vi "test_TCP_TCP Read.vi"(8 "error in (no error)":errorcluster, 11 "TestCase in":refnum<class "Ethernet Protocol Tests.lvclass">) -> (0 "error out":errorcluster, 3 "TestCase out":refnum<class "Ethernet Protocol Tests.lvclass">)   [LabVIEW 2019, in "Ethernet Protocol Tests.lvclass"]
uses:
  Ethernet Protocol Tests.lvclass
  ListenerVi/TCP/TCP.lvclass
  D:/GitRepository/niveristand-instrument-addon-classes/Source/Protocols/Tests/ListenerVi/Protocol Parent/Protocol Parent.lvclass
  ListenerVi/Listener.lvclass
  ListenerVi/TCP/TCP.lvclass/TCP.ctl
  ListenerVi/ListenerClassControls/Operation Ctl.ctl
  ListenerVi/Protocol Parent/Methods/Read Parameter.ctl
  <vilib>/addons/_JKI Toolkits/VI Tester/TestCase.llb/TestCase.lvclass
  ListenerVi/Protocol Parent/Protocol Parent.lvclass
  C:/Program Files (x86)/National Instruments/LabVIEW 2019/vi.lib/addons/_JKI Toolkits/VI Tester/TestCase.llb/TestCase.lvclass
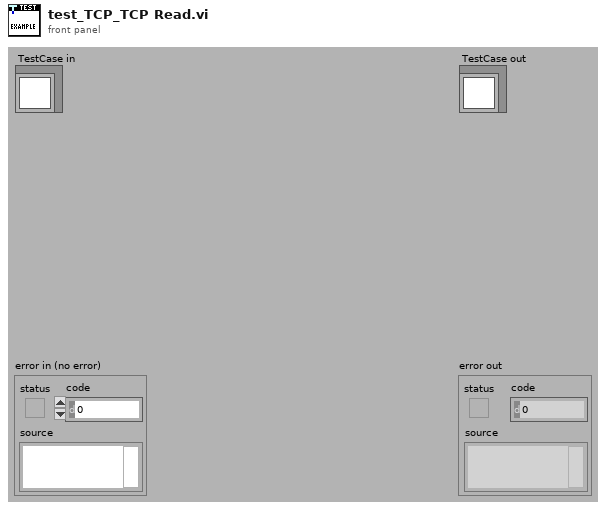
[diagram p1: front panel]
types:
  T1 = typedef "Localhost Protocols.lvlib/Protocol Parent.lvclass/Read Parameter.ctl" = cluster{"Wait Type":enum16{"Byte Count", "Wait sec"}, "Wait Value":dbl}
  T2 = typedef "Operation Ctl.ctl" = enum16{"Read", "Write"}
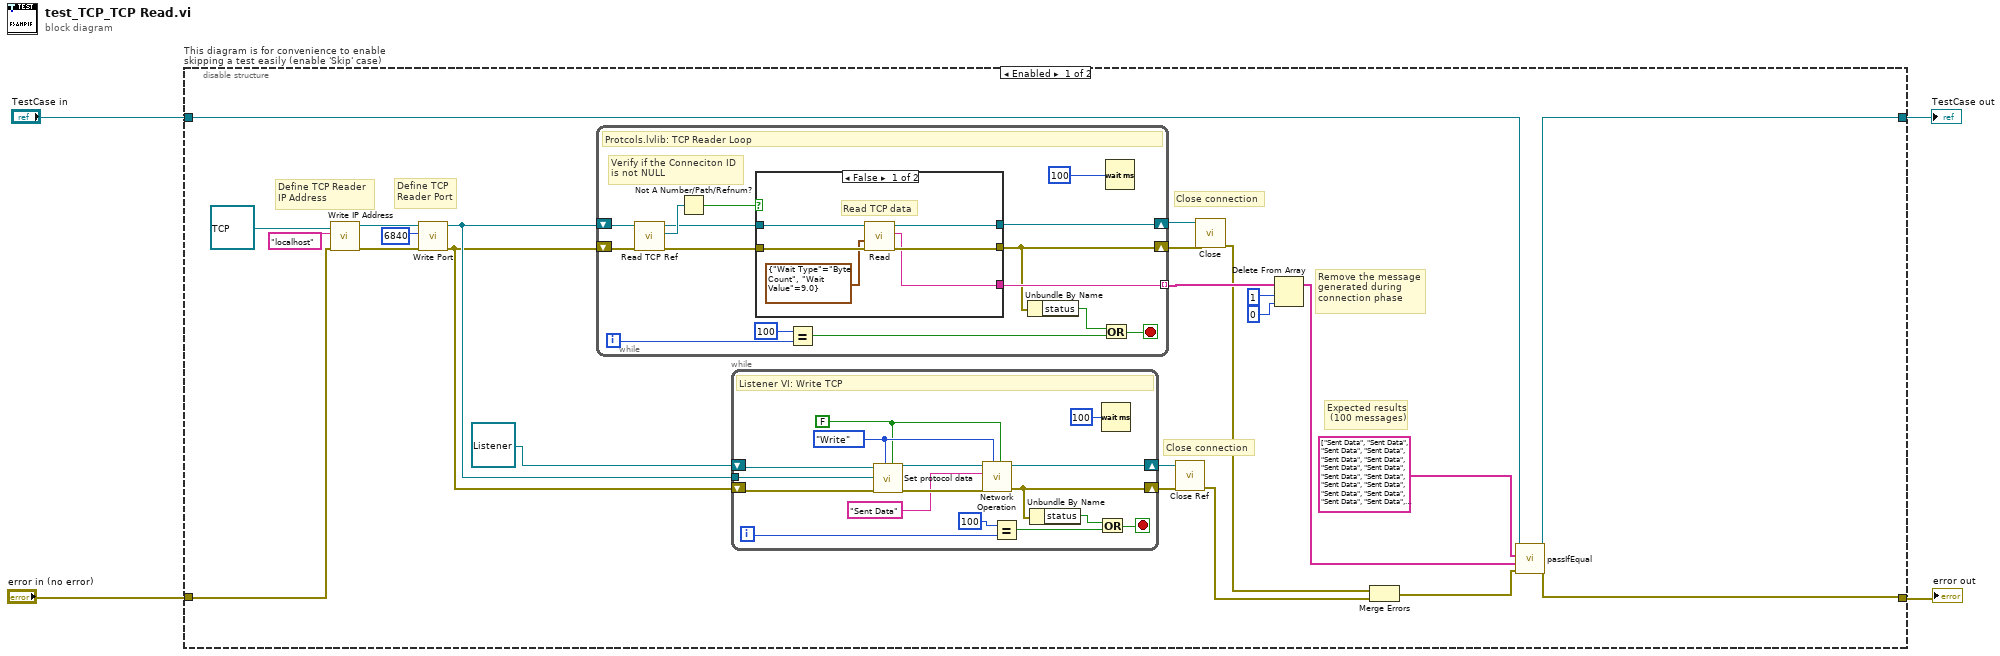
[diagram p0: block diagram]
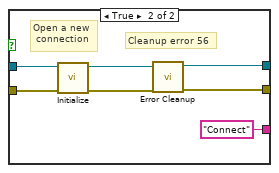
[diagram p2: hidden frame]
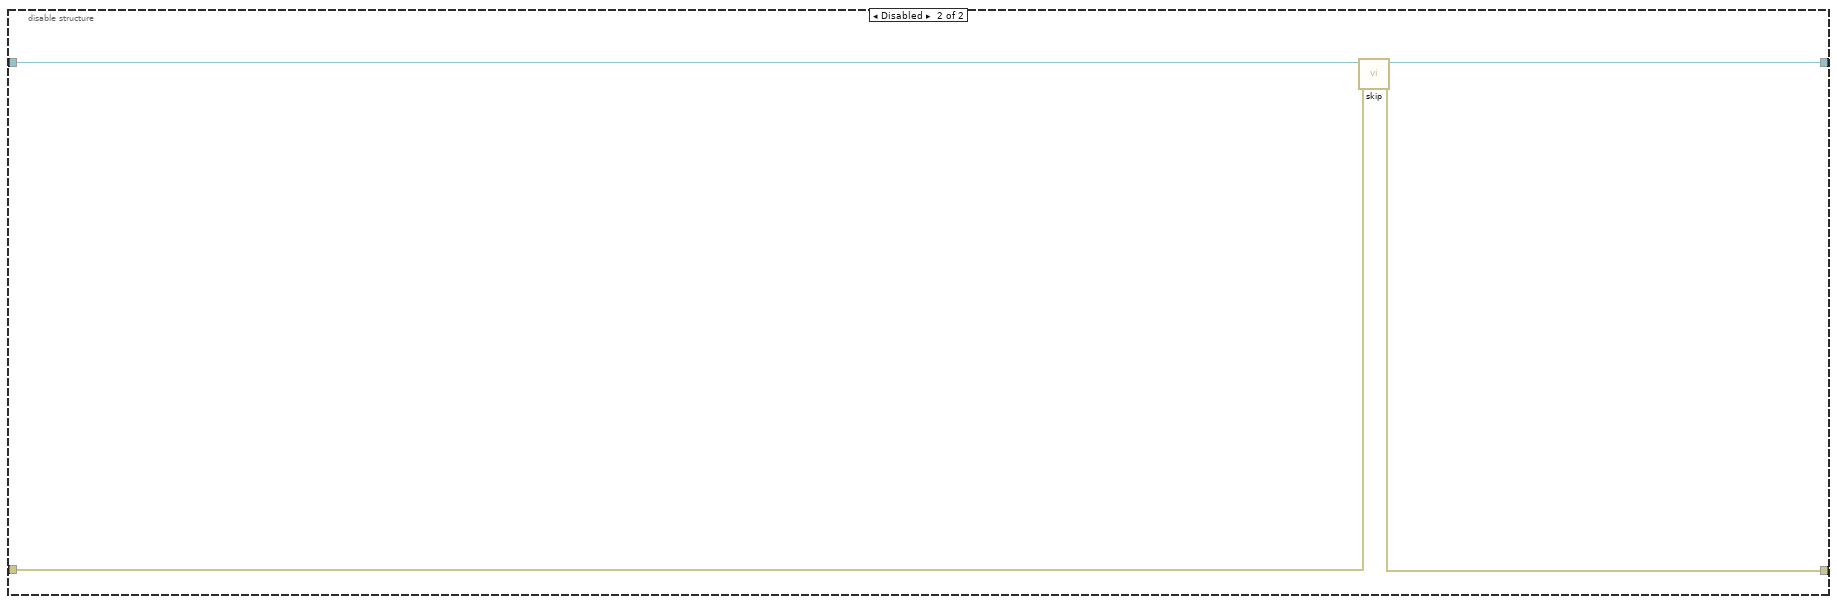
[diagram p3: hidden frame]
diagram:
  n1 = disable-structure "This diagram is for convenience to enable skipping a test easily (enable 'Skip' case)" shown="Enabled" {
    disable-tunnel: "TestCase in" -> [w28 w76]
    disable-tunnel: [w27 w74] -> w1
    disable-tunnel: [w26 w75] -> w3
    disable-tunnel: "error in (no error)" -> [w17 w73]
    frame Enabled {
      # "Close connection"
      # "Close connection"
      # "Remove the message\ngenerated during \nconnection phase"
      # "Expected results\n (100 messages)"
      # "Define TCP \nReader Port"
      # "Define TCP Reader \nIP Address"
      n2 = call "Write IP Address.vi"("error in (no error)"=w17, "IP Address"="localhost", "Ethernet in"=refnum<class "TCP.lvclass"> refnum ("Localhost Protocols.lvlib:TCP.lvclass")) -> ("error out"=w22:errorcluster, "Ethernet out"=w23:refnum<class "TCP.lvclass">)  [unwired: 7 in]
      n3 = call "Write Port.vi"("error in (no error)"=w22, "Port"=u16 6840, "Ethernet in"=w23) -> ("error out"=w18:errorcluster, "Ethernet out"=w20:refnum<class "TCP.lvclass">)  [unwired: 7 in]
      n4 = while {
        shift-right: [w49] -> w10
        shift-left: w18 -> [w59]
        shift-right: [w53] -> w9
        shift-left: w20 -> [w58]
        tunnel: [w52] -> w14 mode=indexing
        i -> [w51]
        stop <- w46 stop-if-true
        # "Verify if the Conneciton ID\nis not NULL"
        # "Protcols.lvlib: TCP Reader Loop"
        n5 = call "Read TCP Ref.vi"("error in (no error)"=w59, "Ethernet in"=w58) -> ("error out"=w54:errorcluster, "TCP Ref"=w57:refnum<k5>, "Ethernet out"=w55:refnum<class "TCP.lvclass">)  [unwired: 7 in]
        n6 = Not A Number/Path/Refnum?(number/path/refnum=w57) -> (NaN/Path/Refnum?=w56:bool)
        n7 = case shown="False" w56 {
          tunnel: w55 -> [w62 w71]
          tunnel: w54 -> [w65 w72]
          tunnel: [w64 w68] -> w49
          tunnel: [w63 w67] -> w53
          tunnel: [w60 "Connect" ("String")] -> w52
          frame False {
            # "Read TCP data"
            n8 = call-dynamic "Read.vi"("error in (no error)"=w65, "Variant"=T1 {"Wait Type"=enum."Byte Count", "Wait Value"=9.0} ("Read Parameter"), "Ethernet in"=w62) -> ("error out"=w64:errorcluster, "String"=w60:string, "Ethernet out"=w63:refnum<class "TCP.lvclass">)  [unwired: 6 in]
          }
          frame True {
            # "Cleanup error 56"
            # "Open a new\n connection"
            n9 = call-dynamic "Initialize.vi"("error in (no error)"=w72, "Ethernet in"=w71) -> ("error out"=w70:errorcluster, "Ethernet out"=w69:refnum<class "TCP.lvclass">)  [unwired: 8 in]
            n10 = call-dynamic "Error Cleanup.vi"("error in (no error)"=w70, "Ethernet in"=w69) -> ("error out"=w68:errorcluster, "Ethernet out"=w67:refnum<class "TCP.lvclass">)  [unwired: 8 in]
          }
        }
        n11 = Equal?(x=100, y=w51) -> (x = y?=w47:bool)
        n12 = Unbundle By Name(w49) -> ("status"=w48:bool)
        n13 = Or(x=w48, y=w47) -> (x .or. y?=w46:bool)
        n14 = Wait (ms)(milliseconds to wait=u32 100) -> ()  [unwired: 1 out]
      }
      n15 = while {
        tunnel: w20 -> [w43]
        shift-right: [w32] -> w6
        shift-left: w18 -> [w44]
        shift-right: [w31] -> w7
        shift-left: refnum<class "Listener.lvclass"> refnum ("Listener.lvclass") -> [w42]
        i -> [w35]
        stop <- w36 stop-if-true
        w38 = FALSE ("AK?")
        w39 = Operation_Ctl."Write" ("Operation")
        # "Listener VI: Write TCP"
        n16 = call "Set protocol data.vi"("AK?"=w38, "Operation"=w39, "error in (no error)"=w44, "Localhost Protocols.lvlib:Protocol Parent.lvclass"=w43, "Listener In.lvclass"=w42) -> ("error out"=w41:errorcluster, "Listener Out.lvclass"=w40:refnum<class "Listener.lvclass">)  [unwired: 5 in]
        n17 = call "Network Operation.vi"("AK?"=w38, "Operation"=w39, "error in (no error)"=w41, "Message"="Sent Data", "Listener In.lvclass"=w40) -> ("error out"=w32:errorcluster, "Listener Out.lvclass"=w31:refnum<class "Listener.lvclass">)  [unwired: 5 in]
        n18 = Equal?(x=100, y=w35) -> (x = y?=w33:bool)
        n19 = Unbundle By Name(w32) -> ("status"=w37:bool)
        n20 = Or(x=w37, y=w33) -> (x .or. y?=w36:bool)
        n21 = Wait (ms)(milliseconds to wait=u32 100) -> ()  [unwired: 1 out]
      }
      n22 = call "Close Ref.vi"("error in (no error)"=w6, "Listener In.lvclass"=w7) -> ("error out"=w5:errorcluster)  [unwired: 9 in]
      n23 = call-dynamic "Close.vi"("error in (no error)"=w10, "Ethernet in"=w9) -> ("error out"=w8:errorcluster)  [unwired: 8 in, 1 out]
      n24 = Delete From Array(array=w14, length=1 ("index"), index=0 ("length")) -> (array with subset deleted=w11:string[])  [unwired: 1 out]
      n25 = Merge Errors(w8, w5) -> (w16:errorcluster)
      n26 = call-dynamic "passIfEqual.vi"("error in (no error)"=w16, "y"=w11, "x"=string[] ["Sent Data", "Sent Data", "Sent Data", "Sent Data", "Sent Data", "Sent Data", "Sent Data", "Sent Data", "Sent Data", "Sent Data", "Sent Data", "Sent Data", "Sent Data", "Sent Data", "Sent Data", "Sent Data", "Sent Data", "Sent Data", "Sent Data", "Sent Data", "Sent Data", "Sent Data", "Sent Data", "Sent Data", "Sent Data", "Sent Data", "Sent Data", "Sent Data", "Sent Data", "Sent Data", "Sent Data", "Sent Data", "Sent Data", "Sent Data", "Sent Data", "Sent Data", "Sent Data", "Sent Data", "Sent Data", "Sent Data", "Sent Data", "Sent Data", "Sent Data", "Sent Data", "Sent Data", "Sent Data", "Sent Data", "Sent Data", "Sent Data", "Sent Data", "Sent Data", "Sent Data", "Sent Data", "Sent Data", "Sent Data", "Sent Data", "Sent Data", "Sent Data", "Sent Data", "Sent Data", "Sent Data", "Sent Data", "Sent Data", "Sent Data", "Sent Data", "Sent Data", "Sent Data", "Sent Data", "Sent Data", "Sent Data", "Sent Data", "Sent Data", "Sent Data", "Sent Data", "Sent Data", "Sent Data", "Sent Data", "Sent Data", "Sent Data", "Sent Data", "Sent Data", "Sent Data", "Sent Data", "Sent Data", "Sent Data", "Sent Data", "Sent Data", "Sent Data", "Sent Data", "Sent Data", "Sent Data", "Sent Data", "Sent Data", "Sent Data", "Sent Data", "Sent Data", "Sent Data", "Sent Data", "Sent Data", "Sent Data"] ("Array"), "TestCase in"=w28) -> ("error out"=w26:errorcluster, "TestCase out"=w27:refnum<class "Ethernet Protocol Tests.lvclass">)  [unwired: 6 in]
    }
    frame Disabled {
      # "skip test result while test is under development"
      n27 = call <vilib>:"skip.vi"("error in (no error)"=w73, "TestCase in"=w76) -> ("error out"=w75:errorcluster, "TestCase out"=w74:refnum<class "Ethernet Protocol Tests.lvclass">)  [unwired: 8 in]
    }
  }
  "error out" <- w3
  "TestCase out" <- w1
